vi "_waveformToDocument.vi"(8 "error in (no error)":errorcluster, 11 "waveform":waveform(dbl)) -> (0 "error out":errorcluster, 3 "tBSONDocument out":refnum<class "tBSONDocument.lvclass">)   [LabVIEW 2013, in "BSON.lvlib" / "tBSONDocument.lvclass"]
doc: "Converts a LabVIEW waveform into a BSON document."
uses:
  tBSONDocument.lvclass
  addTimestampElement.vi
  addDoubleElement.vi
  addDouble[]Element.vi
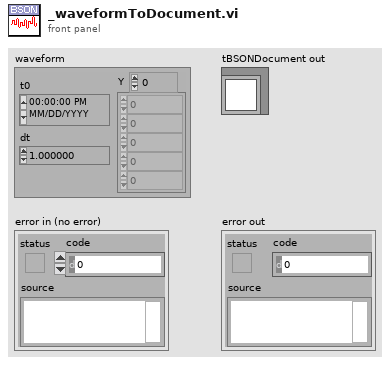
[diagram p1: front panel]
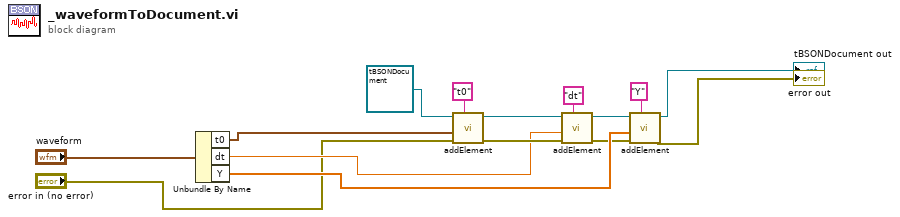
[diagram p0: block diagram]
diagram:
  n1 = Unbundle By Name("waveform") -> ("t0"=w4:timestamp, "dt"=w8:dbl, "Y"=w13:dbl[])
  n2 = call-poly "addElement.vi"("Name"="t0", "error in (no error)"="error in (no error)", "Value"=w4, "tBSONDocument in"=refnum<class "tBSONDocument.lvclass"> refnum ("lvMongoDriver.lvlib:BSON.lvlib:tBSONDocument.lvclass")) -> ("error out"=w9:errorcluster, "tBSONDocument out"=w7:refnum<class "tBSONDocument.lvclass">)  [unwired: 6 in]
  n3 = call-poly "addElement.vi"("Name"="dt", "error in (no error)"=w9, "Value"=w8, "tBSONDocument in"=w7) -> ("error out"=w11:errorcluster, "tBSONDocument out"=w10:refnum<class "tBSONDocument.lvclass">)  [unwired: 6 in]
  n4 = call-poly "addElement.vi"("Name"="Y", "error in (no error)"=w11, "Value"=w13, "tBSONDocument in"=w10) -> ("error out"=→"error out":errorcluster, "tBSONDocument out"=→"tBSONDocument out":refnum<class "tBSONDocument.lvclass">)  [unwired: 6 in]
